vi "WTO.vi"(0 "System no.":i32=1 min=1 max=4 step=1, 2 "Axis to command":string, 3 "No. of output points":i16, 5 "error in":errorcluster, 6 "With Internal Trigger Timer?":bool, 7 "Timer (ms)":i16=1000) -> (19 "error out":errorcluster)   [LabVIEW 2020]
doc: "Sets the wave table output. If No. of output points = 0, wave table output is disabled, otherwise No. of output points will be sent to the given axis. No. of output points must be less than or equal to 64. If With Internal Trigger Timer? is TRUE and Timer (ms) is greater than zero, the internal trigger is used additionally to the external trigger line (if any), but the external trigger resets the internal trigger timer."
panel:
  # "Sets wave table output. If \"No. of output points\" = 0,  wave table\noutput is disabled, otherwise \"No. of output points\" will be sent\nto the given axis. \"No. of output points\" must be less than or\nequal to 64. If With Internal Trigger Timer? is TRUE and Timer \n(ms) is greater than zero, the internal trigger is used additionally\nto the external trigger line (if any), but the external trigger resets\nthe internal trigger timer."
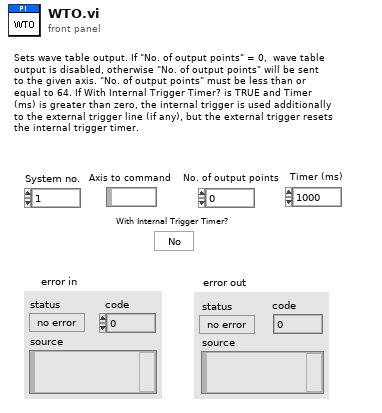
[diagram p1: front panel]
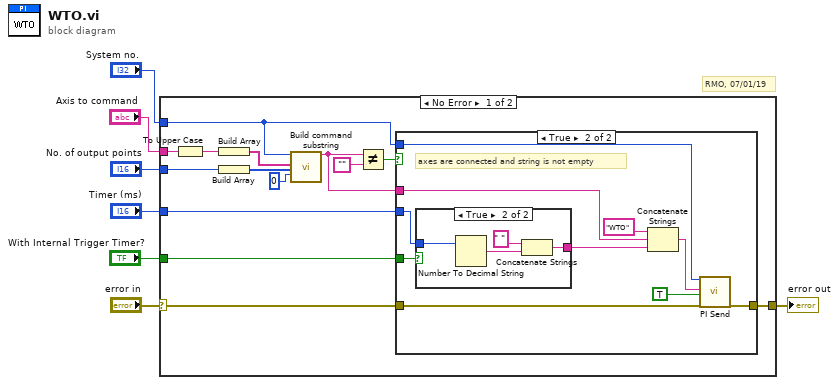
[diagram p0: block diagram]
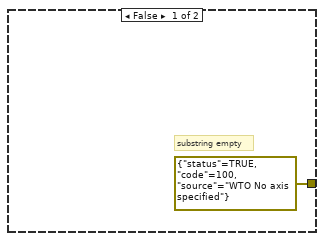
[diagram p2: hidden frame]
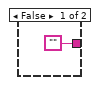
[diagram p3: hidden frame]
diagram:
  # "RMO, 07/01/19"
  n1 = case shown="No Error" "error in" {
    selector: "error in" -> [w8 w38]
    tunnel: [w21 w38] -> w7
    tunnel: "System no." -> [w12 _]
    tunnel: "No. of output points" -> [w16 _]
    tunnel: "Axis to command" -> [w14 _]
    tunnel: "With Internal Trigger Timer?" -> [w11 _]
    tunnel: "Timer (ms)" -> [w10 _]
    frame No Error {
      n2 = To Upper Case(1:w14) -> (0:w13:string)
      n3 = Build Array(w13) -> (w17:string[])
      n4 = Build Array(w16) -> (w15:i16[])
      n5 = call "Build command substring.vi"("System no."=w12, "Affected axes"=w17, "Parameters"=w15, "No. of digits"=i16 0) -> ("Command substring"=w19:string)  [unwired: 3 in, 12 out]
      n6 = Not Equal?(x=w19, y="") -> (x != y?=w9:bool)
      n7 = case shown="True" w9 {
        tunnel: w19 -> [_ w31]
        tunnel: [errorcluster {"status"=TRUE, "code"=100, "source"="WTO No axis specified"} ("error out") w27] -> w21
        tunnel: w8 -> [_ w28]
        tunnel: w12 -> [_ w26]
        tunnel: w11 -> [_ w25]
        tunnel: w10 -> [_ w23]
        frame False {
          # "substring empty"
        }
        frame True {
          # "axes are connected and string is not empty"
          n8 = case shown="True" w25 {
            tunnel: ["" w34] -> w24
            tunnel: w23 -> [_ w37]
            frame False {
            }
            frame True {
              n9 = Number To Decimal String(number=w37) -> (decimal integer string=w36:string)  [unwired: 1 out]
              n10 = Concatenate Strings(" " ("string"), w36) -> (w34:string)
            }
          }
          n11 = Concatenate Strings("WTO", w31, w24) -> (w29:string)
          n12 = call "PI Send.vi"("System no."=w26, "String to send"=w29, "Attach termination char.?"=TRUE ("Attach Linefeed?"), "error in"=w28) -> ("error out"=w27:errorcluster)  [unwired: 2 in, 13 out]
        }
      }
    }
    frame Error {
    }
  }
  "error out" <- w7
